vi "FT10_FPGA_7854R_Main.vi"(0 "75kHz":bool, 5 "uSec On":u16, 7 "uSec Off":u16, 9 "Conn2/DIO_0_7 In":bool[](array[boolean])=[FALSE, FALSE, FALSE, FALSE, FALSE, FALSE, FALSE, FALSE], 11 "Conn2/DIO_8_15 In":bool[](array[boolean])=[FALSE, FALSE, FALSE, FALSE, FALSE, FALSE, FALSE, FALSE]) -> (10 "Conn2/DIO_0_7 Out":bool[](array[boolean]), 15 "Conn2/DIO_8_15 Out":bool[](array[boolean]))   [LabVIEW 2015]
doc: "This VI defines the BitFile loaded onto the NI PXI-7854R Module"
uses:
  <vilib>/eio/EIONode/EIONode.xnode
  <vilib>/rvi/eio/common/nirviEmuTemplateMethod_errors.vi
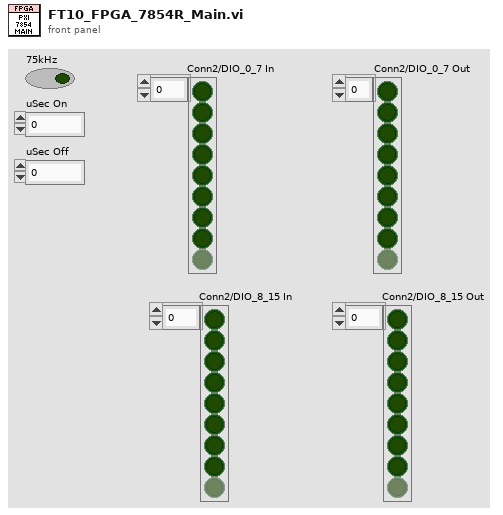
[diagram p1: front panel]
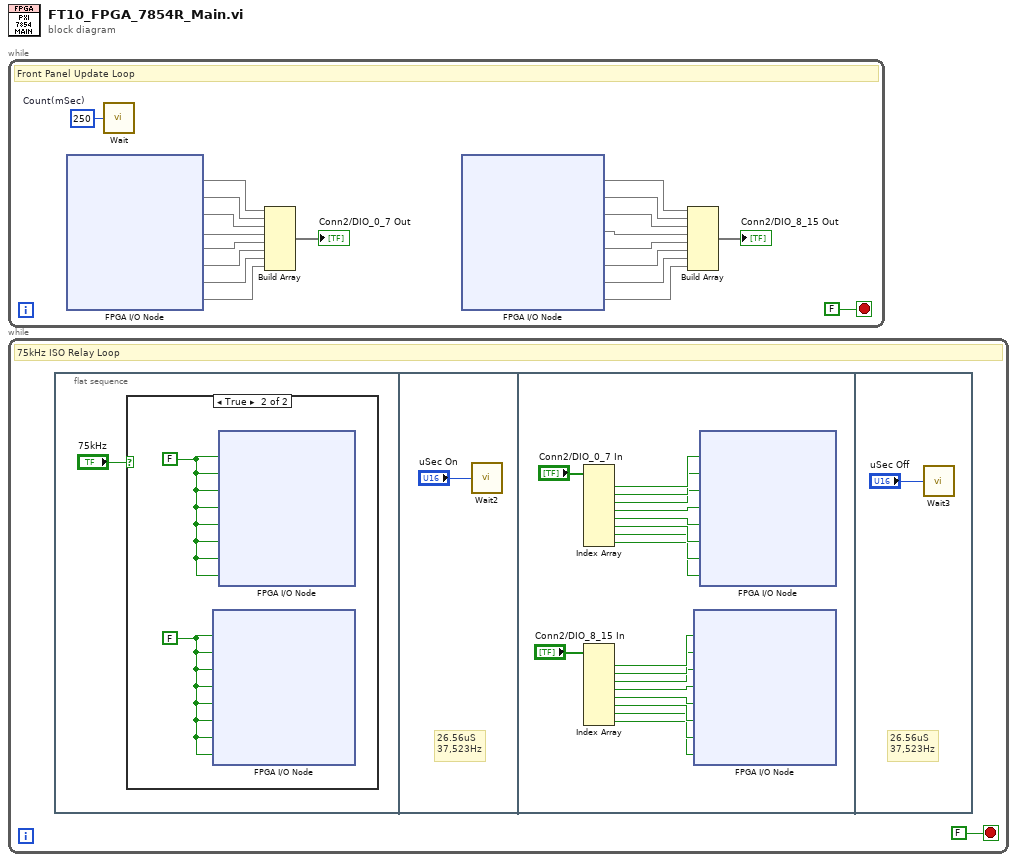
[diagram p0: block diagram]
diagram:
  n1 = while {
    stop <- FALSE stop-if-true
    w19 = u8 250  # Count(mSec)
    # "Front Panel Update Loop"
    n2 = xnode "FPGA I/O Node"() -> ("Connector2/DIO0"=w18, "Connector2/DIO1"=w17, "Connector2/DIO2"=w16, "Connector2/DIO3"=w15, "Connector2/DIO4"=w14, "Connector2/DIO5"=w13, "Connector2/DIO6"=w12, "Connector2/DIO7"=w11)  [unwired: 8 in, 8 out]
    n3 = call "Wait"("Count(mSec)"=w19) -> ()  [unwired: 1 out]
    n4 = Build Array(w18, w17, w16, w15, w14, w13, w12, w11) -> (→"Conn2/DIO_0_7 Out":void[])
    n5 = xnode "FPGA I/O Node"() -> ("Connector2/DIO8"=w9, "Connector2/DIO9"=w8, "Connector2/DIO10"=w7, "Connector2/DIO11"=w6, "Connector2/DIO12"=w5, "Connector2/DIO13"=w4, "Connector2/DIO14"=w3, "Connector2/DIO15"=w2)  [unwired: 8 in, 8 out]
    n6 = Build Array(w9, w8, w7, w6, w5, w4, w3, w2) -> (→"Conn2/DIO_8_15 Out":void[])
  }
  n7 = while {
    stop <- FALSE stop-if-true
    # "75kHz ISO Relay Loop"
    n8 = flat-sequence {
      frame #0 {
        n9 = case shown="True" "75kHz" {
          frame False {
          }
          frame True {
            w24 = FALSE ("Connector2/DIO8")
            w23 = FALSE ("Connector2/DIO0")
            n10 = xnode "FPGA I/O Node"("Connector2/DIO8"=w24, "Connector2/DIO9"=w24, "Connector2/DIO10"=w24, "Connector2/DIO11"=w24, "Connector2/DIO12"=w24, "Connector2/DIO13"=w24, "Connector2/DIO14"=w24, "Connector2/DIO15"=w24) -> ()  [unwired: 8 in, 8 out]
            n11 = xnode "FPGA I/O Node"("Connector2/DIO0"=w23, "Connector2/DIO1"=w23, "Connector2/DIO2"=w23, "Connector2/DIO3"=w23, "Connector2/DIO4"=w23, "Connector2/DIO5"=w23, "Connector2/DIO6"=w23, "Connector2/DIO7"=w23) -> ()  [unwired: 8 in, 8 out]
          }
        }
      }
      frame #1 {
        # "26.56uS\n37,523Hz"
        n12 = call "Wait2"("Count(uSec)"="uSec On") -> ()  [unwired: 1 out]
      }
      frame #2 {
        n13 = Index Array(array="Conn2/DIO_0_7 In") -> (element #1=w41:bool, element #2=w40:bool, element #3=w39:bool, element #4=w38:bool, element #5=w37:bool, element #6=w36:bool, element #7=w35:bool, element #8=w34:bool)  [unwired: 8 in]
        n14 = Index Array(array="Conn2/DIO_8_15 In") -> (element #1=w33:bool, element #2=w32:bool, element #3=w31:bool, element #4=w30:bool, element #5=w29:bool, element #6=w28:bool, element #7=w27:bool, element #8=w26:bool)  [unwired: 8 in]
        n15 = xnode "FPGA I/O Node"("Connector2/DIO8"=w33, "Connector2/DIO9"=w32, "Connector2/DIO10"=w31, "Connector2/DIO11"=w30, "Connector2/DIO12"=w29, "Connector2/DIO13"=w28, "Connector2/DIO14"=w27, "Connector2/DIO15"=w26) -> ()  [unwired: 8 in, 8 out]
        n16 = xnode "FPGA I/O Node"("Connector2/DIO0"=w41, "Connector2/DIO1"=w40, "Connector2/DIO2"=w39, "Connector2/DIO3"=w38, "Connector2/DIO4"=w37, "Connector2/DIO5"=w36, "Connector2/DIO6"=w35, "Connector2/DIO7"=w34) -> ()  [unwired: 8 in, 8 out]
      }
      frame #3 {
        # "26.56uS\n37,523Hz"
        n17 = call "Wait3"("Count(uSec)"="uSec Off") -> ()  [unwired: 1 out]
      }
    }
  }
